vi "sub_process channels.vi"   [LabVIEW 2021]
uses:
  <vilib>/Utility/file.llb/Read Delimited Spreadsheet (I64).vi
  <vilib>/Utility/file.llb/Read Delimited Spreadsheet (string).vi
  <vilib>/Utility/file.llb/Read Delimited Spreadsheet (DBL).vi
  globalvariables.vi
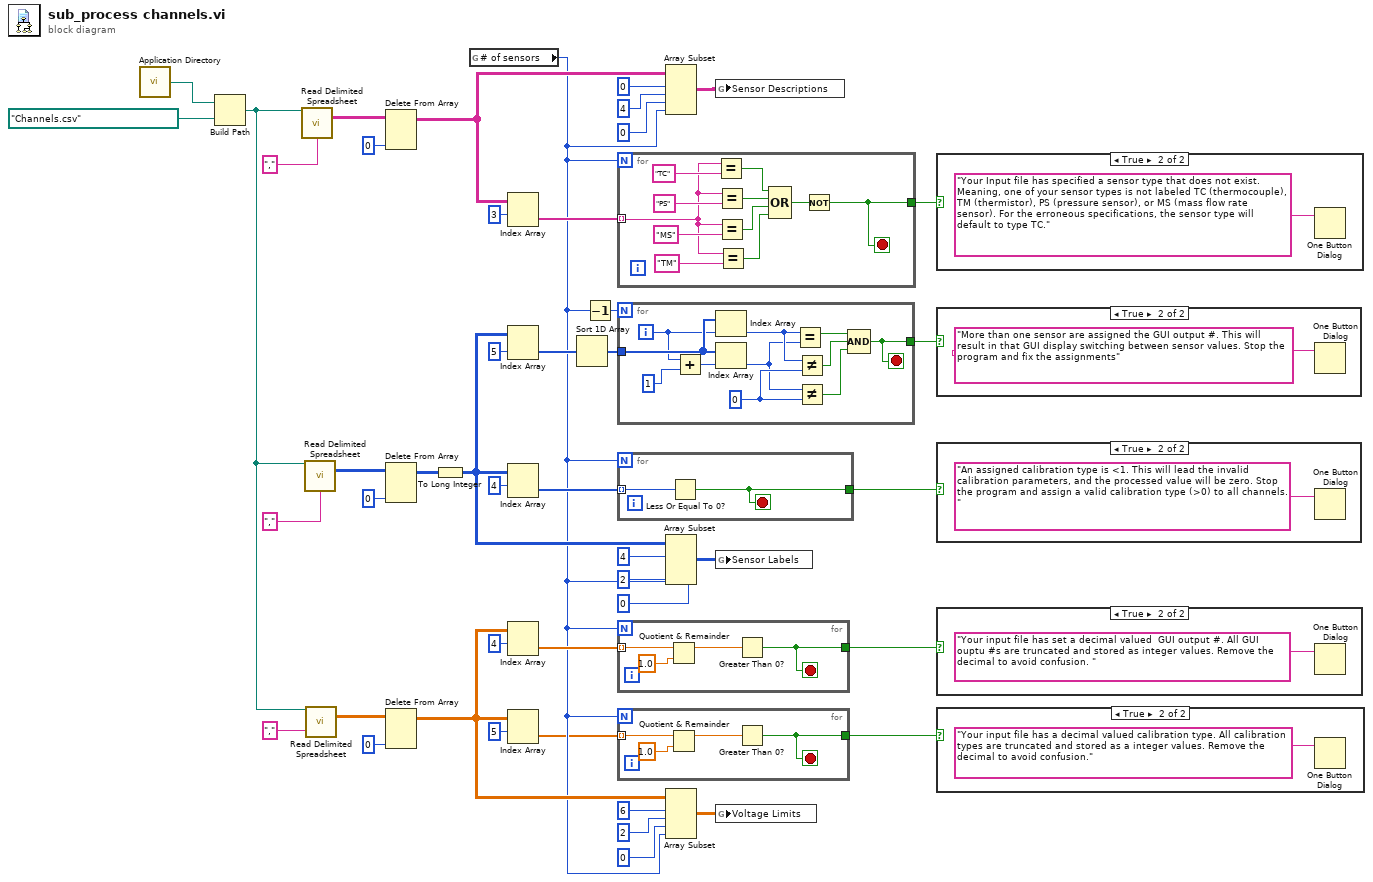
[diagram p0: block diagram]
diagram:
  n1 = call <vilib>:"Application Directory.vi"() -> ("Application Directory"=w30:path)
  n2 = Build Path(base path=w30, name or relative path=path "Channels.csv") -> (appended path=w37:path)
  n3 = call-poly <vilib>:"Read Delimited Spreadsheet.vi"("file path (dialog if empty)"=w37, "delimiter (\\t)"=",") -> ("all rows"=w41:string[][])  [unwired: 8 in, 5 out]
  n4 = call-poly <vilib>:"Read Delimited Spreadsheet.vi"("file path (dialog if empty)"=w37, "delimiter (\\t)"=",") -> ("all rows"=w43:i64[][])  [unwired: 8 in, 5 out]
  n5 = call-poly <vilib>:"Read Delimited Spreadsheet.vi"("file path (dialog if empty)"=w37, "delimiter (\\t)"=",") -> ("all rows"=w18:dbl[][])  [unwired: 8 in, 5 out]
  n6 = Delete From Array(array=w41, index (col)=0) -> (array with subset deleted=w15:string[][])  [unwired: 2 in, 1 out]
  n7 = Delete From Array(array=w43, index (col)=0) -> (array with subset deleted=w6:i64[][])  [unwired: 2 in, 1 out]
  n8 = Delete From Array(array=w18, index (col)=0) -> (array with subset deleted=w17:dbl[][])  [unwired: 2 in, 1 out]
  n9 = To Long Integer(number=w6) -> (32bit integer=w5:i32[][])
  n10 = global read "globalvariables.vi" "# of sensors"() -> (w3:i32)
  n11 = Index Array(array=w15, index (row)=3) -> (element=w39:string[])  [unwired: 1 in]
  n12 = Index Array(array=w5, index (row)=5) -> (element=w25:i32[])  [unwired: 1 in]
  n13 = Index Array(array=w5, index (row)=4) -> (element=w28:i32[])  [unwired: 1 in]
  n14 = Index Array(array=w17, index (row)=4) -> (element=w33:dbl[])  [unwired: 1 in]
  n15 = Index Array(array=w17, index (row)=5) -> (element=w2:dbl[])  [unwired: 1 in]
  n16 = Sort 1D Array(array=w25) -> (sorted array=w44:i32[])
  n17 = Decrement(x=w3) -> (x-1=w45:i32)
  n18 = for {
    N: w3 -> [_]
    tunnel: w39 -> [w47] mode=indexing
    tunnel: [w48] -> w40
    stop <- w48 stop-if-true
    n19 = Equal?(x=w47, y="TC") -> (x = y?=w54:bool)
    n20 = Equal?(x=w47, y="PS") -> (x = y?=w53:bool)
    n21 = Equal?(x=w47, y="MS") -> (x = y?=w52:bool)
    n22 = Equal?(x=w47, y="TM") -> (x = y?=w50:bool)
    n23 = Compound Arithmetic op=OR(w54, w53, w52, w50) -> (w49:bool)
    n24 = Not(x=w49) -> (.not. x?=w48:bool)
  }
  n25 = for {
    N: w45 -> [_]
    tunnel: w44 -> [w60]
    tunnel: [w58] -> w46
    i -> [w59]
    stop <- w58 stop-if-true
    w66 = 0
    n26 = Add(x=w59, y=1) -> (x+y=w67:i32)
    n27 = Index Array(array=w60, index=w59) -> (element=w65:i32)
    n28 = Index Array(array=w60, index=w67) -> (element=w64:i32)
    n29 = Equal?(x=w65, y=w64) -> (x = y?=w61:bool)
    n30 = Not Equal?(x=w65, y=w66) -> (x != y?=w63:bool)
    n31 = Not Equal?(x=w64, y=w66) -> (x != y?=w62:bool)
    n32 = Compound Arithmetic op=AND(w61, w63, w62) -> (w58:bool)
  }
  n33 = for {
    N: w3 -> [_]
    tunnel: w28 -> [w69] mode=indexing
    tunnel: [w70] -> w29
    stop <- w70 stop-if-true
    n34 = Less Or Equal To 0?(x=w69) -> (x <= 0?=w70:bool)
  }
  n35 = for {
    N: w3 -> [_]
    tunnel: w33 -> [w72] mode=indexing
    tunnel: [w71] -> w34
    stop <- w71 stop-if-true
    n36 = Quotient & Remainder(x=w72, y=1.0) -> (x-y*floor(x/y)=w73:dbl)  [unwired: 1 out]
    n37 = Greater Than 0?(x=w73) -> (x > 0?=w71:bool)
  }
  n38 = for {
    N: w3 -> [_]
    tunnel: w2 -> [w76] mode=indexing
    tunnel: [w75] -> w1
    stop <- w75 stop-if-true
    n39 = Quotient & Remainder(x=w76, y=1.0) -> (x-y*floor(x/y)=w77:dbl)  [unwired: 1 out]
    n40 = Greater Than 0?(x=w77) -> (x > 0?=w75:bool)
  }
  n41 = Array Subset(array=w15, index (row)=0, length (row)=4, index (col)=0, length (col)=w3) -> (w4:string[][])
  n42 = Array Subset(array=w5, index (row)=4, length (row)=2, index (col)=0, length (col)=w3) -> (w7:i32[][])
  n43 = Array Subset(array=w17, index (row)=6, length (row)=2, index (col)=0, length (col)=w3) -> (w8:dbl[][])
  n44 = global write "globalvariables.vi" "Sensor Descriptions"(w4) -> ()
  n45 = global write "globalvariables.vi" "Sensor Labels"(w7) -> ()
  n46 = global write "globalvariables.vi" "Voltage Limits"(w8) -> ()
  n47 = case shown="True" w40 {
    frame False {
    }
    frame True {
      n48 = One Button Dialog(message="Your Input file has specified a sensor type that does not exist. Meaning, one of your sensor types is not labeled TC (thermocouple), TM (thermistor), PS (pressure sensor), or MS (mass flow rate sensor). For the erroneous specifications, the sensor type will default to type TC.") -> ()  [unwired: 1 in, 1 out]
    }
  }
  n49 = case shown="True" w46 {
    frame False {
    }
    frame True {
      n50 = One Button Dialog(message="More than one sensor are assigned the GUI output #. This will result in that GUI display switching between sensor values. Stop the program and fix the assignments") -> ()  [unwired: 1 in, 1 out]
    }
  }
  n51 = case shown="True" w29 {
    frame False {
    }
    frame True {
      n52 = One Button Dialog(message="An assigned calibration type is <1. This will lead the invalid calibration parameters, and the processed value will be zero. Stop the program and assign a valid calibration type (>0) to all channels.") -> ()  [unwired: 1 in, 1 out]
    }
  }
  n53 = case shown="True" w34 {
    frame False {
    }
    frame True {
      n54 = One Button Dialog(message="Your input file has set a decimal valued  GUI output #. All GUI ouptu #s are truncated and stored as integer values. Remove the decimal to avoid confusion. ") -> ()  [unwired: 1 in, 1 out]
    }
  }
  n55 = case shown="True" w1 {
    frame False {
    }
    frame True {
      n56 = One Button Dialog(message="Your input file has a decimal valued calibration type. All calibration types are truncated and stored as a integer values. Remove the decimal to avoid confusion.") -> ()  [unwired: 1 in, 1 out]
    }
  }
